vi "Read Data.vi"(8 "error in (no error)":errorcluster, 11 "Expansion in":refnum<class "Expansion.lvclass">) -> (0 "error out":errorcluster, 2 "Data":variant, 3 "Expansion out":refnum<class "Expansion.lvclass">)   [LabVIEW 2017, in "Expansion.lvclass"]
uses:
  Expansion.lvclass
  Expansion.lvclass/Expansion.ctl
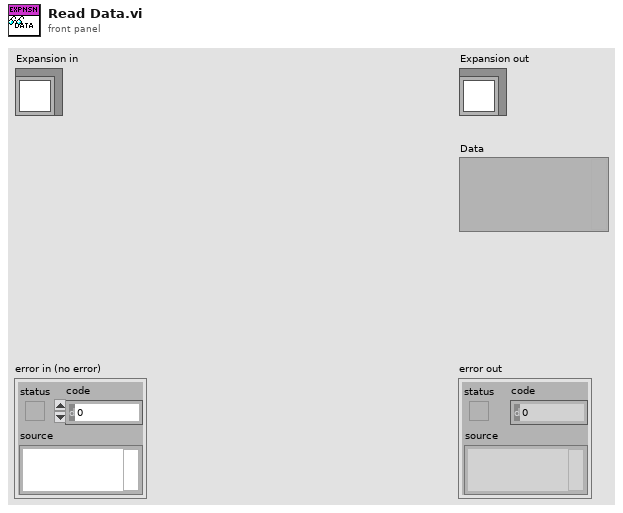
[diagram p1: front panel]
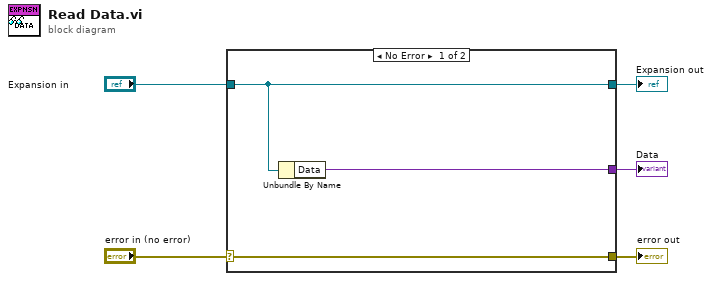
[diagram p0: block diagram]
diagram:
  n1 = case shown="No Error" "error in (no error)" {
    selector: "error in (no error)" -> [w8 w9]
    tunnel: [w8 w9] -> w4
    tunnel: [w7 w10] -> w2
    tunnel: "Expansion in" -> [w7 w10]
    tunnel: [w6 _] -> w1
    frame No Error {
      n2 = Unbundle By Name(w7) -> ("Data"=w6:variant)
    }
    frame Error {
    }
  }
  "error out" <- w4
  "Expansion out" <- w2
  "Data" <- w1
